vi "SVL AC & DC Level (Time) (1 Ch).vi"(0 "scaled signal [EU]":waveform(dbl)={"t0"=timestamp(0 s since 1904-01-01), "dt"=0.0, "Y"=[]}, 2 "window":T1=1 items=["None"=0, "Hanning"=1, "Hamming"=2, "Blackman-Harris"=3, "Exact Blackman"=4, "Blackman"=5, "Flat Top"=6, "4 Term B-Harris "=7, "7 Term B-Harris"=8, "Low Sidelobe"=9, "Force"=64, "Exponential"=65, "Blackman Nuttall"=11, "Triangle"=30, "Bartlett-Hanning"=31, "Bohman"=32, "Parzen"=33, "Welch"=34, "Kaiser"=60, "Dolph-Chebyshev"=61, "Gaussian"=62], 5 "error in (no error)":errorcluster) -> (12 "unit label":string, 14 "AC signal [EU]":waveform(dbl), 15 "AC level [EU rms]":dbl=nan format="%.8f", 16 "DC signal [EU]":waveform(dbl), 17 "DC level [EU]":dbl=nan format="%0.2f", 19 "error out":errorcluster)   [LabVIEW 2017]
doc: "Computes the AC level and DC level of a signal. Wire data to the <B>scaled signal [EU]</B> input to determine the polymorphic instance to use or manually select the instance."
uses:
  <vilib>/addons/_NISVFA/_Shared subVIs/Controls/svc_Window.ctl
  <vilib>/Analysis/baseanly.llb/Mean (DBL).vi
  <vilib>/Analysis/4window.llb/Force Window.vi
  <vilib>/Analysis/4window.llb/Force Window (DBL).vi
  <vilib>/Analysis/4window.llb/Exponential Window.vi
  <vilib>/Analysis/4window.llb/Exponential Window (DBL).vi
  <vilib>/Utility/error.llb/Error Cluster From Error Code.vi
  <vilib>/Analysis/0measdsp.llb/Scaled Time Domain Window.vi
  <vilib>/Analysis/0measdsp.llb/Scaled Time Domain Window (DBL).vi
  <vilib>/addons/_NISVFA/_Spectrum Processing/subVIs/svfa_Spectrum Info Window to windowTd Type Def.vi
  <vilib>/addons/_NISVFA/_Shared subVIs/Common/svc_Engineering Units to Unit Label.vi
  <vilib>/addons/_NISVFA/_Shared subVIs/Common/svc_Unit Label to Engineering Units.vi
  <vilib>/Analysis/NI_AALBase.lvlib
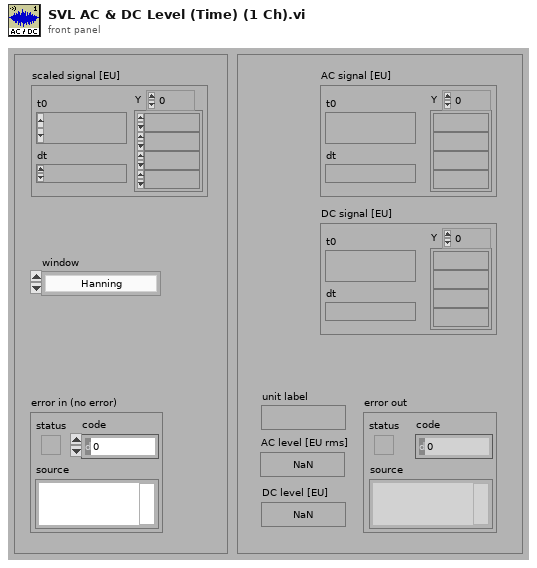
[diagram p1: front panel]
types:
  T1 = typedef "svc_Window.ctl" = u32
  T2 = typedef "NI_AALPro.lvlib/windowTd.ctl" = u32
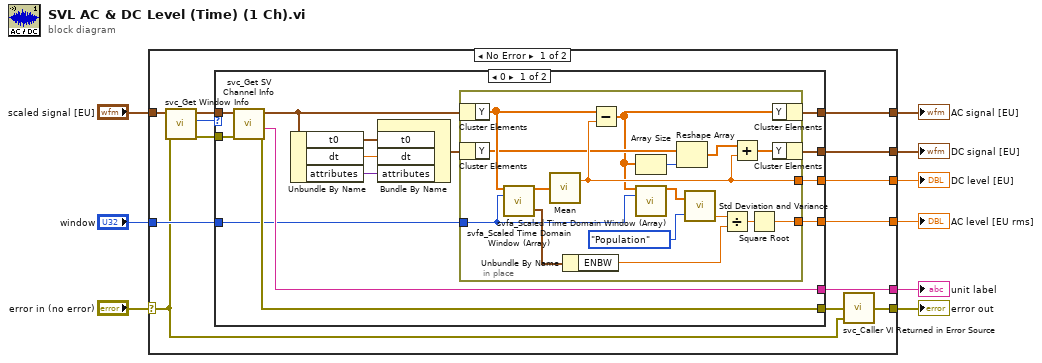
[diagram p0: block diagram]
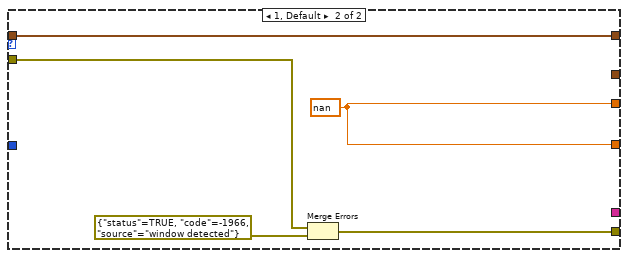
[diagram p2: hidden frame]
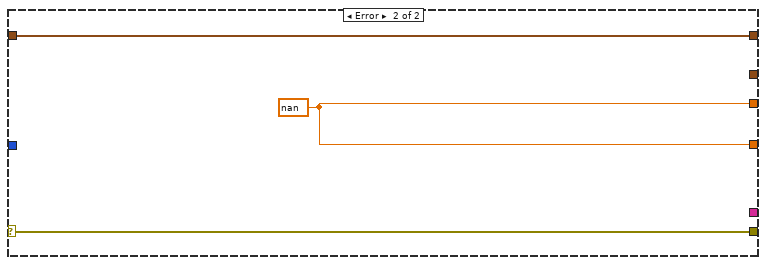
[diagram p3: hidden frame]
diagram:
  n1 = case shown="No Error" "error in (no error)" {
    selector: "error in (no error)" -> [w12 w60]
    tunnel: [w22 w59] -> w9
    tunnel: "window" -> [w17 _]
    tunnel: [w16 w58] -> w7
    tunnel: "scaled signal [EU]" -> [w15 w58]
    tunnel: [w21 w59] -> w5
    tunnel: [w18 w60] -> w3
    tunnel: [w20 _] -> w2
    tunnel: [w10 _] -> w1
    frame No Error {
      n2 = call <vilib>:"svc_Get Window Info.vi"("error in (no error)"=w12, "scaled signal [EU]"=w15) -> ("error out"=w13:errorcluster, "window"=w11:T2, "dup scaled signal [EU]"=w14:waveform(dbl))  [unwired: 5 in, 2 out]
      n3 = case shown="0" w11 {
        tunnel: [w31 w54] -> w22
        tunnel: [w30 w54] -> w21
        tunnel: [w34 _] -> w20
        tunnel: [w33 w57] -> w19
        tunnel: w17 -> [w32 _]
        tunnel: [w29 w53] -> w16
        tunnel: w14 -> [w36 w53]
        tunnel: w13 -> [w35 w56]
        tunnel: [w23 _] -> w10
        frame 0 {
          n4 = call <vilib>:"svc_Get SV Channel Info.vi"("error in (no error)"=w35, "scaled signal [EU]"=w36) -> ("error out"=w33:errorcluster, "unit label"=w34:string, "dup scaled signal [EU]"=w27:waveform(dbl))  [unwired: 4 in, 3 out]
          n5 = Unbundle By Name(w27) -> ("t0"=w26:timestamp, "dt"=w25:dbl, "attributes"=w24:variant)
          n6 = Bundle By Name("t0"=w26, "dt"=w25, "attributes"=w24) -> (w28:waveform(dbl))  [unwired: 1 in]
          n7 = in-place {
            in-place-border: [w44] -> w30
            in-place-border: w32 -> [w45]
            in-place-border: [w46] -> w31
            n8 = in-place-cluster #1(w27) -> ("Y"=w51:dbl[])
            n9 = in-place-cluster #2(w28) -> ("Y"=w40:dbl[])
            n10 = call <vilib>:"svfa_Scaled Time Domain Window (Array).vi"("input signal"=w51, "window"=w45) -> ("windowed signal"=w42:dbl[], "window constants"=w52:cluster{"ENBW":dbl, "CG":dbl})  [unwired: 8 in, 4 out]
            n11 = call-poly <vilib>:"Mean.vi"("X"=w42) -> ("mean"=w44:dbl)  [unwired: 1 out]
            n12 = Unbundle By Name(w52) -> ("ENBW"=w47:dbl)
            n13 = Subtract(x=w51, y=w44) -> (x-y=w38:dbl[])
            n14 = Array Size(array=w38) -> (size(s)=w39:i32)
            n15 = call <vilib>:"svfa_Scaled Time Domain Window (Array).vi"("input signal"=w38, "window"=w45) -> ("windowed signal"=w41:dbl[])  [unwired: 8 in, 5 out]
            n16 = Reshape Array(w40, w39) -> (w37:dbl[])
            n17 = call <vilib>:"Std Deviation and Variance.vi"("X"=w41, "Weighting (Sample)"=enum16{"Sample", "Population"}."Population") -> ("variance"=w50:dbl)  [unwired: 2 out]
            n18 = Divide(x=w50, y=w47) -> (x/y=w48:dbl)
            n19 = Add(x=w37, y=w44) -> (x+y=w43:dbl[])
            n20 = Square Root(x=w48) -> (sqrt(x)=w46:dbl)
            n21 = in-place-cluster #1("Y"=w38) -> (w29:waveform(dbl))
            n22 = in-place-cluster #2("Y"=w43) -> (w23:waveform(dbl))
          }
        }
        frame 1, Default {
          w54 = nan ("mean")
          n23 = Merge Errors(w56, errorcluster {"status"=TRUE, "code"=-1966, "source"="window detected"} ("error in 2 (no error)")) -> (w57:errorcluster)
        }
      }
      n24 = call <vilib>:"svc_Caller VI Returned in Error Source.vi"("warning input to caller"=w12, "error in (no error)"=w19) -> ("error out"=w18:errorcluster)  [unwired: 3 in]
    }
    frame Error {
      w59 = nan
    }
  }
  "AC level [EU rms]" <- w9
  "DC level [EU]" <- w5
  "AC signal [EU]" <- w7
  "error out" <- w3
  "unit label" <- w2
  "DC signal [EU]" <- w1
